vi "Frame_to_word_14444B UP.vi"() -> ()   [LabVIEW 2019]
uses:
  <vilib>/addons/Modulation/Analog/MT Modulate AM (DSB).vi
  <vilib>/addons/Modulation/Analog/MT Upconvert Baseband (Real).vi
  <vilib>/express/express analysis/Spectral/Block/exnSpectralBlock spectral measurements RMS poly.vi
  <vilib>/express/express analysis/Spectral/Block/exnSpectralBlock spectral measurements RMS WFM.vi
  <vilib>/ErrorRing/Error Ring.xnode
  <vilib>/express/express analysis/Spectral/XNode/ExpressSpectralMeasurementsBlockNode.xnode
  <vilib>/addons/Modulation/niAMT.lvlib
panel:
  out "video Manchecter 8":cluster{"t0":dbl, "dt":dbl, "Y":dbl[]}(graph)
  out "video Manchecter 2":cluster{"t0":dbl, "dt":dbl, "Y":dbl[]}(graph)
  out "video Manchecter 7":waveform(dbl)(graph)
  out "video Manchecter 6":cluster{"t0":dbl, "dt":dbl, "Y":dbl[]}(graph)
  out "video Manchecter 5":waveform(dbl)(graph)
  out "video Manchecter 4":cluster{"t0":dbl, "dt":dbl, "Y":dbl[]}(graph)
  out "video Manchecter":cluster{"t0":dbl, "dt":dbl, "Y":dbl[]}(graph)
  in  "BIT RATE":dbl
  in  "CARRIER (hz)":dbl=1356000.0
  out "Video  without CRC":cluster{"t0":dbl, "dt":dbl, "Y":dbl[]}(graph)
  out "Video":cluster{"t0":dbl, "dt":dbl, "Y":dbl[]}(graph)
  in  "1":u8[](array[numeric])=[80] format="%x"
  in  "PUPI":u8[](array[numeric])=[178, 212, 178, 212] format="%x"
  in  "Protocol Info":u8[](array[numeric])=[3, 33, 227] format="%x"
  in  "App data":u8[](array[numeric])=[213, 18, 68, 243] format="%x"
  # "App data"
  # "Protocol info"
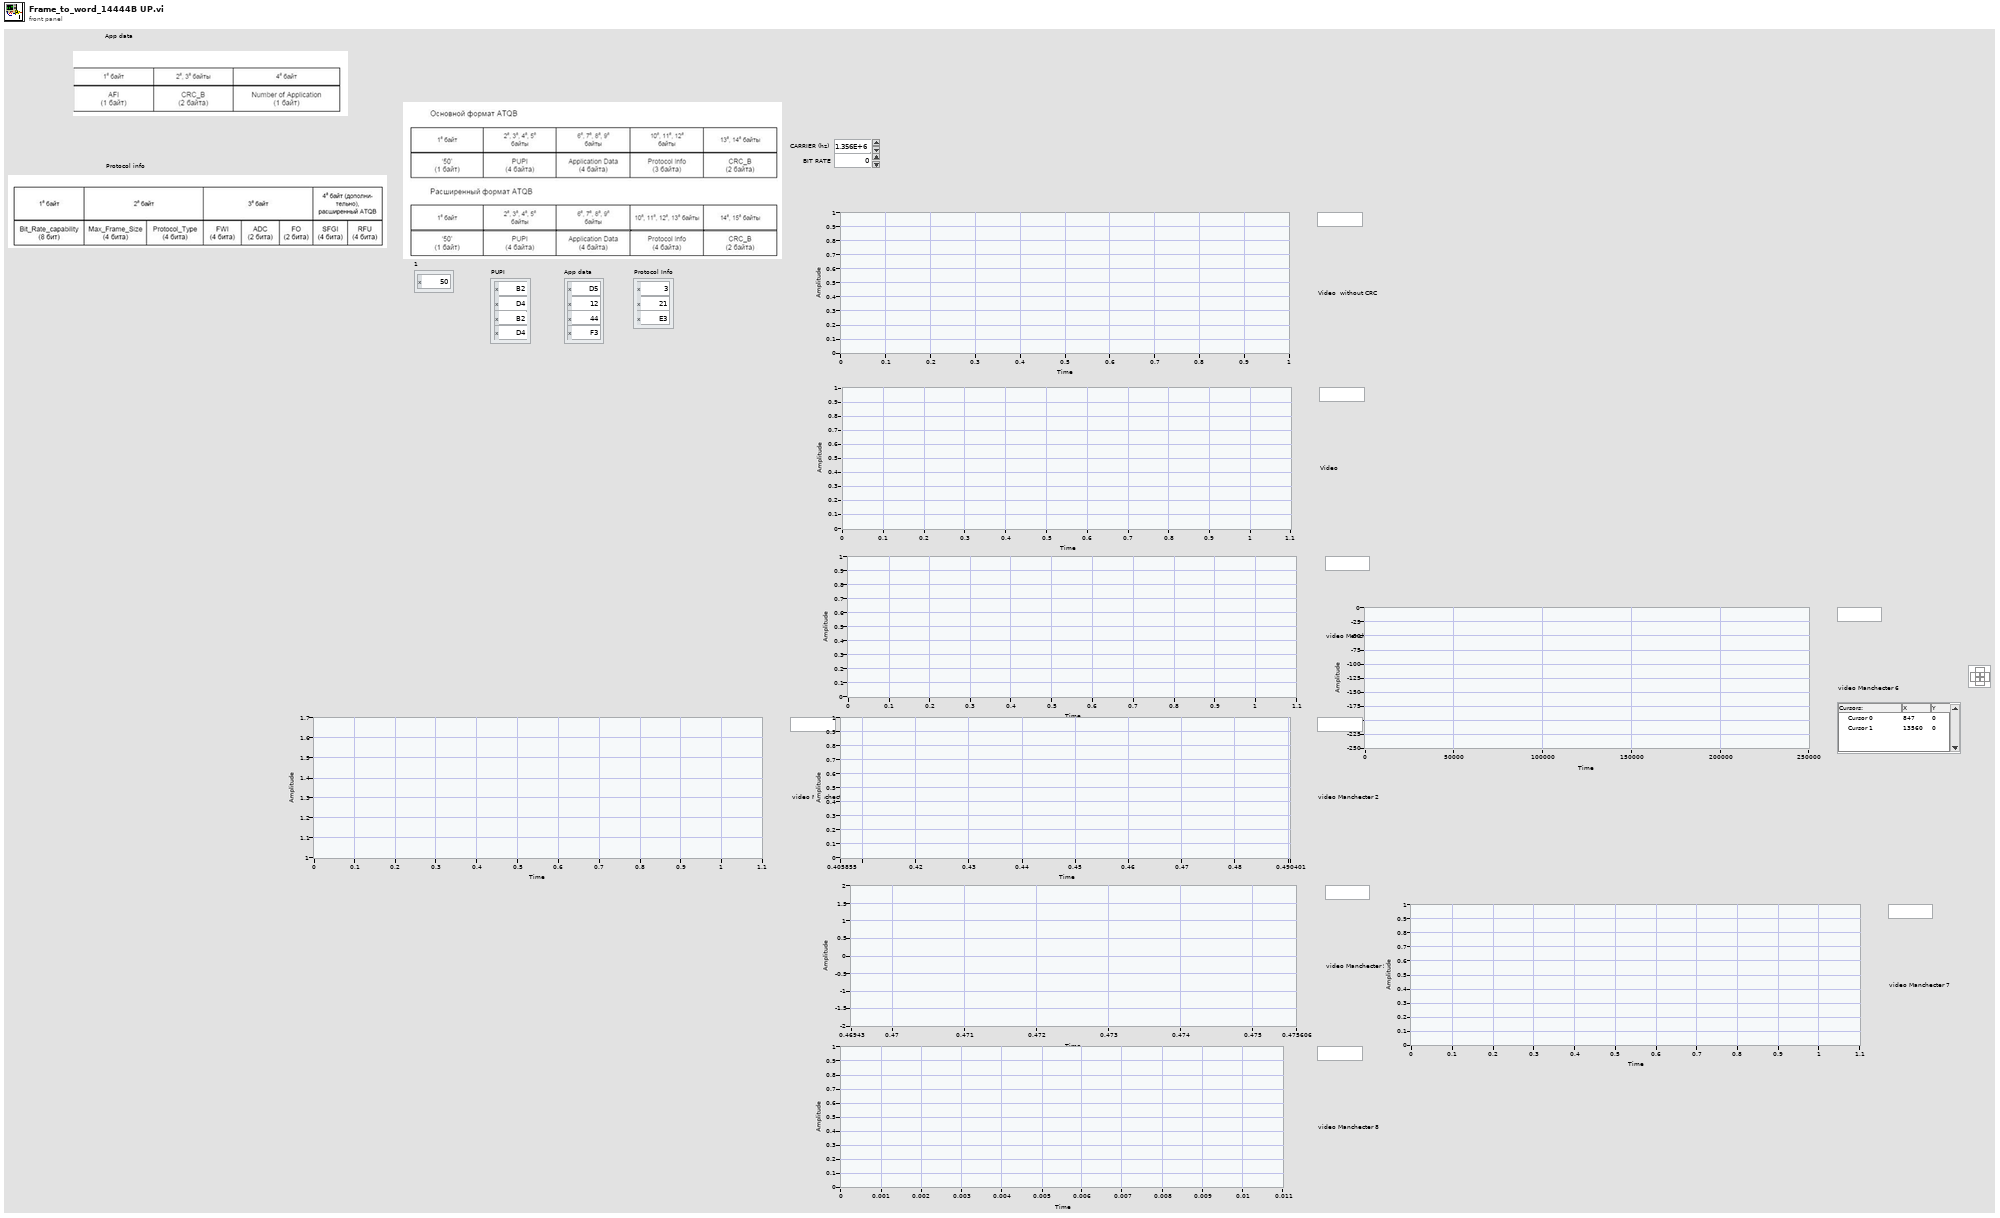
[diagram p1: front panel]
types:
  T1 = typedef "niAMT.lvlib/Complex Data Waveform.ctl" = cluster{"t0":dbl, "dt":dbl, "Y":cdb[]}
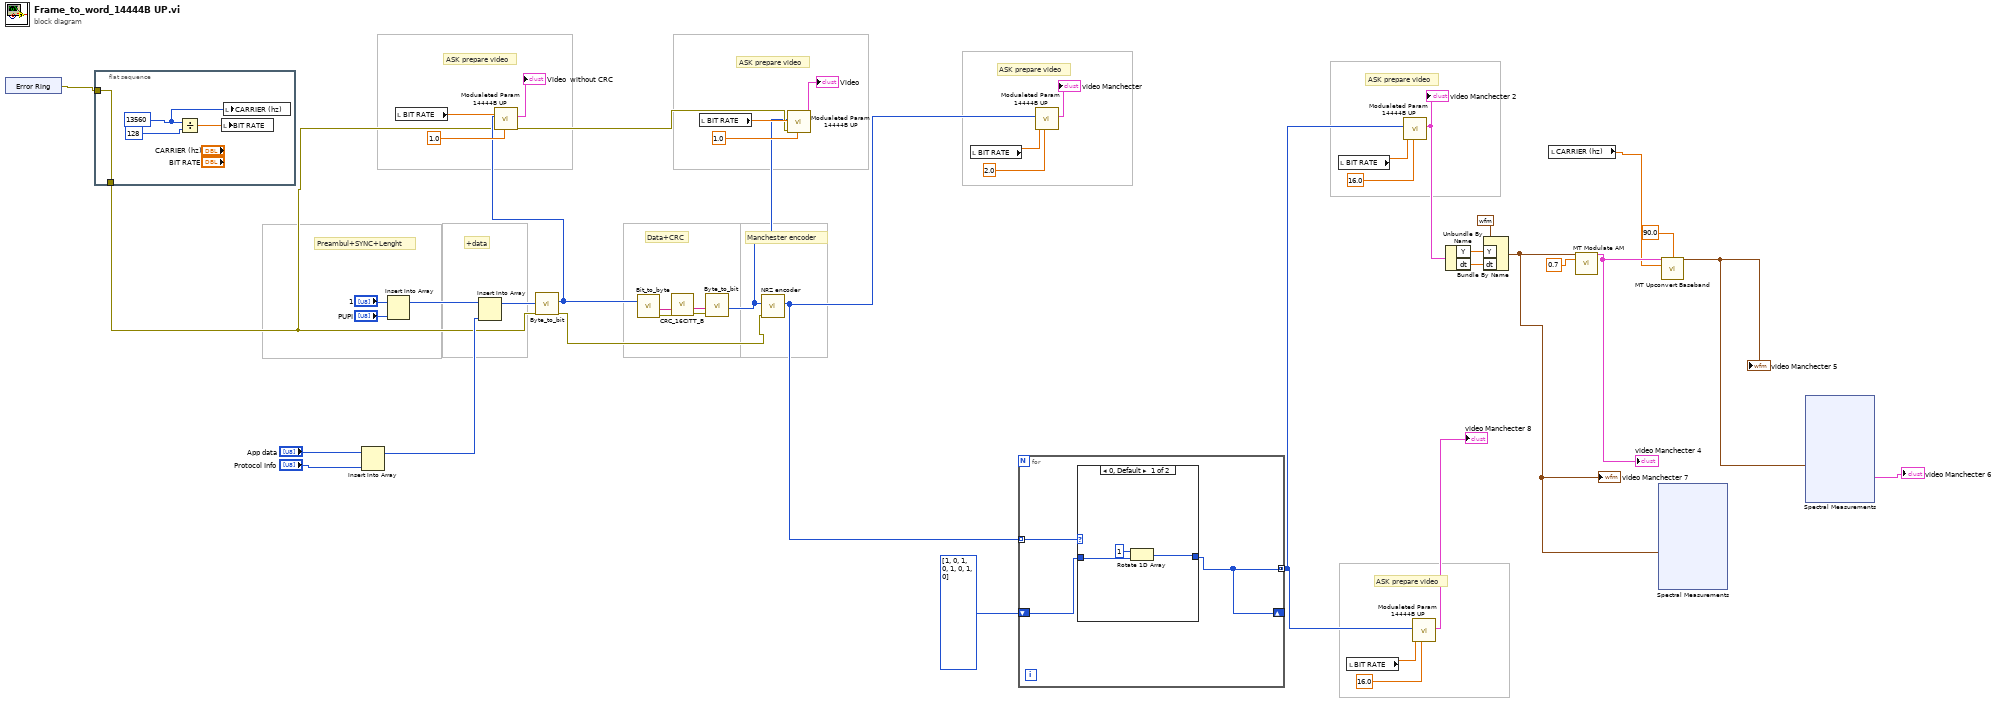
[diagram p0: block diagram]
diagram:
  (unwired) 16.0 ("y")
  # "ASK prepare video"
  # "ASK prepare video"
  # "ASK prepare video"
  # "ASK prepare video"
  # "ASK prepare video"
  # "ASK prepare video"
  # "Manchester encoder"
  # "Data+CRC"
  # "+data"
  # "Preambul+SYNC+Lenght"
  n1 = xnode "Error Ring"() -> ("error out"=w31:errorcluster)
  n2 = flat-sequence {
    tunnel: w31 -> [w46]
    tunnel: [w46] -> w30
    frame #0 {
      w47 = u32 13560
      n3 = Divide(x=w47, y=u32 128) -> (x/y=w48:dbl)
      n4 = local write "BIT RATE"(w48) -> ()
      n5 = local write "CARRIER (hz)"(w47) -> ()
    }
  }
  n6 = Insert Into Array(array="App data", new element="Protocol Info") -> (w41:u8[])  [unwired: 1 in]
  n7 = Insert Into Array(array="1", new element="PUPI") -> (w40:u8[])  [unwired: 1 in]
  n8 = local read "BIT RATE"() -> (w34:dbl)
  n9 = Insert Into Array(array=w40, new element=w41) -> (w33:u8[])  [unwired: 1 in]
  n10 = call "Byte_to_bit.vi"("Error In"=w30, "Array of byte"=w33) -> ("Error Out"=w13:errorcluster, "Arrray of bit"=w32:u8[])  [unwired: 5 in, 1 out]
  n11 = call "Modualeted Param 14444B UP.vi"("encoder divider"=1.0 ("y"), "Error In"=w30, "BIT RATE"=w34, "Bit stream out (NRZ encode)"=w32) -> ("Error Out"=w29:errorcluster, "output complex waveform"=→"Video  without CRC":T1)  [unwired: 6 in]
  n12 = call "Bit_to_byte.vi"("Array of bit"=w32) -> ("Error Out"=w4:errorcluster, "BYTE"=w3:string)  [unwired: 8 in, 1 out]
  n13 = call "CRC_16CITT_B.vi"("Error In"=w4, "DATA PACKET"=w3) -> ("Error Out"=w2:errorcluster, "DATA PACKET+CRC"=w1:string)  [unwired: 5 in, 1 out]
  n14 = local read "BIT RATE"() -> (w39:dbl)
  n15 = call "Byte_to_bit.vi"("Error In"=w2, "BYTE"=w1) -> ("Arrray of bit (str)"=w14:u8[])  [unwired: 5 in, 2 out]
  n16 = call "NRZ encoder.vi"("Error In"=w13, "Bit stream in"=w14) -> ("Bit stream out (NRZ encode)"=w8:u8[])  [unwired: 8 in, 1 out]
  n17 = call "Modualeted Param 14444B UP.vi"("encoder divider"=1.0 ("y"), "Error In"=w29, "BIT RATE"=w39, "Bit stream out (NRZ encode)"=w14) -> ("output complex waveform"=→"Video":T1)  [unwired: 6 in, 1 out]
  n18 = local read "BIT RATE"() -> (w27:dbl)
  n19 = for {
    tunnel: w8 -> [w52] mode=indexing
    tunnel: [w50] -> w7 mode=concatenating
    shift-right: [w50] -> _
    shift-left: u8[] [1, 0, 1, 0, 1, 0, 1, 0] ("output array") -> [w51]
    n20 = case shown="0, Default" w52 {
      tunnel: w51 -> [w55 w56]
      tunnel: [w54 w56] -> w50
      frame 0, Default {
        n21 = Rotate 1D Array(1:w55, 2:1 ("n")) -> (0:w54:u8[])
      }
      frame 1 {
      }
    }
  }
  n22 = call "Modualeted Param 14444B UP.vi"("encoder divider"=2.0 ("y"), "BIT RATE"=w27, "Bit stream out (NRZ encode)"=w8) -> ("output complex waveform"=→"video Manchecter":T1)  [unwired: 7 in, 1 out]
  n23 = local read "BIT RATE"() -> (w25:dbl)
  n24 = local read "BIT RATE"() -> (w17:dbl)
  n25 = call "Modualeted Param 14444B UP.vi"("encoder divider"=16.0 ("y"), "BIT RATE"=w25, "Bit stream out (NRZ encode)"=w7) -> ("output complex waveform"=w10:T1)  [unwired: 7 in, 1 out]
  "video Manchecter 2" <- w10
  n26 = call "Modualeted Param 14444B UP.vi"("encoder divider"=16.0 ("y"), "BIT RATE"=w17, "Bit stream out (NRZ encode)"=w7) -> ("output complex waveform"=→"video Manchecter 8":T1)  [unwired: 7 in, 1 out]
  n27 = Unbundle By Name(w10) -> ("Y"=w20:cdb[], "dt"=w19:dbl)
  n28 = Bundle By Name(cluster=waveform(cdb) {"t0"=timestamp(0 s since 1904-01-01), "dt"=1.0, "Y"=[]} ("waveform"), "Y"=w20, "dt"=w19) -> (w18:waveform(cdb))
  "video Manchecter 7" <- w18
  n29 = local read "CARRIER (hz)"() -> (w5:dbl)
  n30 = call-poly <vilib>:"MT Modulate AM.vi"("message signal"=w18, "modulation index"=0.7) -> ("AM modulated waveform"=w22:cluster{"t0":dbl, "dt":dbl, "Y":cdb[]})  [unwired: 12 in, 1 out]
  "video Manchecter 4" <- w22
  n31 = xnode "Spectral Measurements"("Signals"=w18) -> ()  [unwired: 1 in, 3 out]
  n32 = call-poly <vilib>:"MT Upconvert Baseband.vi"("baseband waveform (complex)"=w22, "initial phase (deg)"=90.0, "carrier frequency (Hz)"=w5) -> ("passband waveform"=w9:waveform(dbl))  [unwired: 11 in, 1 out]
  "video Manchecter 5" <- w9
  n33 = xnode "Spectral Measurements"("Signals"=w9) -> ("FFT - (RMS)"=→"video Manchecter 6":cluster{"f0":dbl, "df":dbl, "magnitude":dbl[]})  [unwired: 1 in, 2 out]
